vi "FramelessFP Drop-In.vi"(8 "error in (no error)":errorcluster, 11 "Pane in":refnum<vi>) -> (0 "error out":errorcluster)   [LabVIEW 2019]
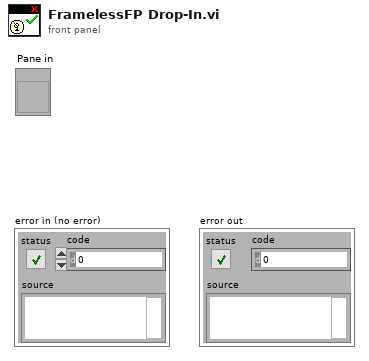
[diagram p1: front panel]
types:
  T1 = cluster{"OwningVI":refnum<vi>, "device ID":refnum<k1>}
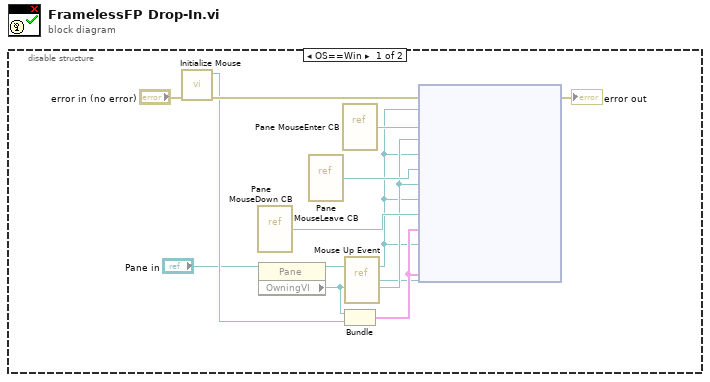
[diagram p0: block diagram]
diagram:
  n1 = disable-structure shown="OS==Win" {
    frame condition #0 {
      n2 = call <vilib>:"Initialize Mouse.vi"("error in (no error)"="error in (no error)") -> ("error out"=w10:errorcluster, "device ID"=w7:refnum<k1>)  [unwired: 9 in]
      n3 = vi-ref "Pane MouseDown CB.vi"() -> ("vi reference"=w8:refnum<vi>)
      n4 = property class="Pane"(reference="Pane in") -> (reference out=w1:refnum<vi>, "OwningVI"=w4:refnum<vi>)  [unwired: 1 in, 1 out]
      n5 = vi-ref "Pane MouseLeave CB.vi"() -> ("vi reference"=w6:refnum<vi>)
      n6 = vi-ref "Pane MouseEnter CB.vi"() -> ("vi reference"=w9:refnum<vi>)
      n7 = vi-ref "Mouse Up Event.vi"() -> ("vi reference"=w2:refnum<vi>)
      n8 = Bundle("OwningVI"=w4, "device ID"=w7) -> (w3:T1)  [unwired: 1 in]
      n9 = node(w10, w1, w9, w4, w1, w6, w4, w1, w8, w3, w1, w2, w3) -> (→"error out":errorcluster)  [unwired: 1 in, 1 out]
    }
    frame condition #1 (active) {
    }
  }
